vi "convert_FIFO_data_USB7855R.vi"(0 "Actual Data":i16[](array[numeric]), 5 "Calinbration Costants":cluster{"LSB Weight":u32, "Offset":i32}[](array[cluster])) -> (19 "appended array":dbl[][](array[numeric]))   [LabVIEW 2023]
uses:
  User_Vi/Settings.vi
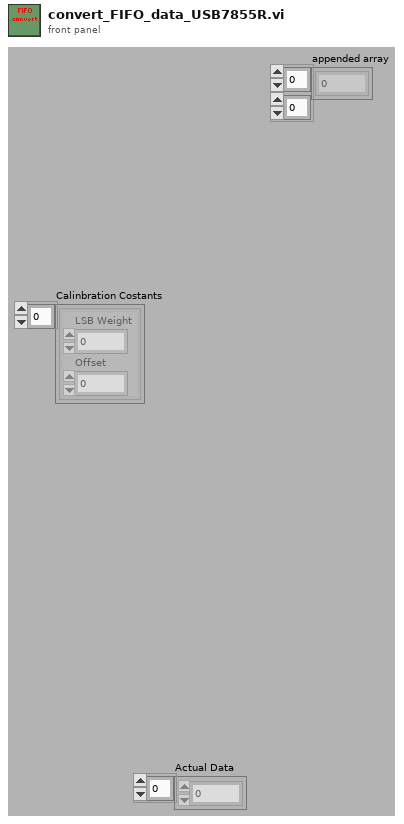
[diagram p1: front panel]
types:
  T1 = typedef "Current Amplifier Settings.ctl" = dbl
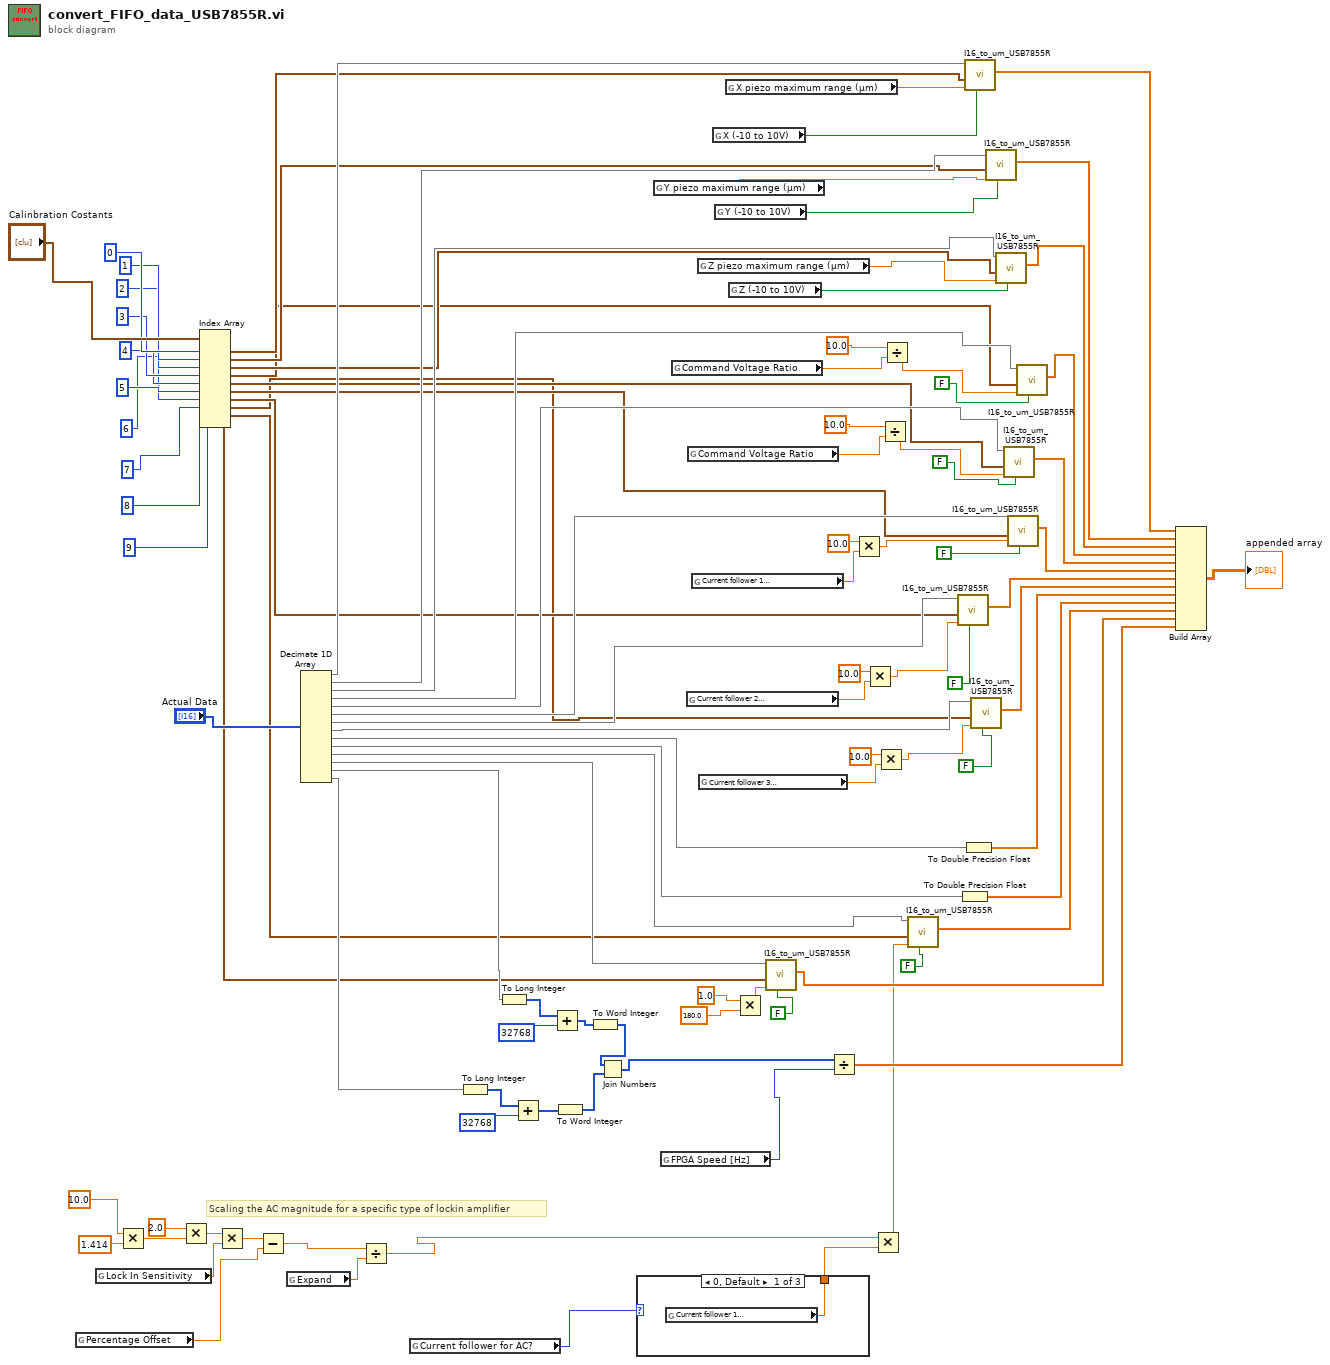
[diagram p0: block diagram]
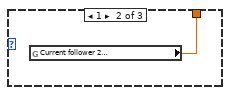
[diagram p2: hidden frame]
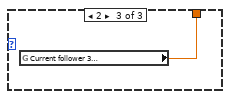
[diagram p3: hidden frame]
diagram:
  # "Scaling the AC magnitude for a specific type of lockin amplifier"
  n1 = global read "Settings.vi" "Percentage Offset"() -> (w33:dbl)
  n2 = global read "Settings.vi" "Lock In Sensitivity"() -> (w31:dbl)
  n3 = Multiply(x=10.0 ("y"), y=1.414) -> (x*y=w25:dbl)
  n4 = Multiply(x=2.0 ("y"), y=w25) -> (x*y=w30:dbl)
  n5 = Index Array(array="Calinbration Costants", index #1=0 ("index"), index #2=1 ("index"), index #3=2 ("index"), index #4=3 ("index"), index #5=4 ("index"), index #6=5 ("index"), index #7=6 ("index"), index #8=7 ("index"), index #9=8 ("index"), index #10=9 ("index")) -> (element #1=w19:cluster{"LSB Weight":u32, "Offset":i32}, element #2=w17:cluster{"LSB Weight":u32, "Offset":i32}, element #3=w10:cluster{"LSB Weight":u32, "Offset":i32}, element #4=w7:cluster{"LSB Weight":u32, "Offset":i32}, element #5=w6:cluster{"LSB Weight":u32, "Offset":i32}, element #6=w5:cluster{"LSB Weight":u32, "Offset":i32}, element #7=w4:cluster{"LSB Weight":u32, "Offset":i32}, element #8=w3:cluster{"LSB Weight":u32, "Offset":i32}, element #9=w2:cluster{"LSB Weight":u32, "Offset":i32}, element #10=w1:cluster{"LSB Weight":u32, "Offset":i32})
  n6 = Multiply(x=w30, y=w31) -> (x*y=w32:dbl)
  n7 = Subtract(x=w32, y=w33) -> (x-y=w27:dbl)
  n8 = global read "Settings.vi" "Expand"() -> (w28:dbl)
  n9 = Decimate 1D Array("Actual Data") -> (w74:i16[], w70:i16[], w64:i16[], w61:i16[], w56:i16[], w53:i16[], w49:i16[], w46:i16[], w95:i16[], w94:i16[], w37:i16[], w42:i16[], w89:i16[], w84:i16[])
  n10 = Divide(x=w27, y=w28) -> (x/y=w29:dbl)
  n11 = global read "Settings.vi" "Current follower for AC?"() -> (w35:u8)
  n12 = To Long Integer(number=w84) -> (32bit integer=w85:i32[])
  n13 = To Long Integer(number=w89) -> (32bit integer=w88:i32[])
  n14 = Add(x=w85, y=32768 ("Max Value [um]")) -> (x+y=w81:i32[])
  n15 = Add(x=w88, y=32768 ("Max Value [um]")) -> (x+y=w82:i32[])
  n16 = To Word Integer(number=w81) -> (16bit integer=w80:i16[])
  n17 = To Word Integer(number=w82) -> (16bit integer=w79:i16[])
  n18 = Join Numbers(hi=w79, lo=w80) -> ((hi.lo)=w83:u32[])
  n19 = case shown="0, Default" w35 {
    tunnel: [w106 w107 w108] -> w34
    frame 0, Default {
      n20 = global read "Settings.vi" "Current follower 1\n (AI-3)"() -> (w106:T1)
    }
    frame 1 {
      n21 = global read "Settings.vi" "Current follower 2 \n(AI-4)"() -> (w107:T1)
    }
    frame 2 {
      n22 = global read "Settings.vi" "Current follower 3\n(AI-6)"() -> (w108:T1)
    }
  }
  n23 = global read "Settings.vi" "Y piezo maximum range (µm)"() -> (w69:dbl)
  n24 = global read "Settings.vi" "FPGA Speed [Hz]"() -> (w77:i64)
  n25 = global read "Settings.vi" "Command Voltage Ratio"() -> (w76:dbl)
  n26 = global read "Settings.vi" "Current follower 2 \n(AI-4)"() -> (w99:T1)
  n27 = global read "Settings.vi" "Command Voltage Ratio"() -> (w75:dbl)
  n28 = global read "Settings.vi" "Current follower 1\n (AI-3)"() -> (w101:T1)
  n29 = global read "Settings.vi" "Z piezo maximum range (µm)"() -> (w63:dbl)
  n30 = global read "Settings.vi" "Current follower 3\n(AI-6)"() -> (w96:T1)
  n31 = global read "Settings.vi" "X (-10 to 10V)"() -> (w72:bool)
  n32 = global read "Settings.vi" "Y (-10 to 10V)"() -> (w68:bool)
  n33 = global read "Settings.vi" "X piezo maximum range (µm)"() -> (w73:dbl)
  n34 = global read "Settings.vi" "Z (-10 to 10V)"() -> (w66:bool)
  n35 = Multiply(x=1.0, y=180.0) -> (x*y=w39:dbl)
  n36 = call "I16_to_um_USB7855R.vi"("-10 to 10V range?"=FALSE, "Max Value [um]"=w39, "Channel Calibration"=w1, "Input_I16"=w42) -> ("output_um"=w41:dbl[])  [unwired: 7 in]
  n37 = Divide(x=w83, y=w77) -> (x/y=w90:dbl[])
  n38 = Multiply(x=10.0 ("Max Value [um]"), y=w101) -> (x*y=w52:T1)
  n39 = Multiply(x=10.0 ("Max Value [um]"), y=w99) -> (x*y=w48:T1)
  n40 = Multiply(x=w29, y=w34) -> (x*y=w23:T1)
  n41 = Multiply(x=10.0 ("Max Value [um]"), y=w96) -> (x*y=w43:T1)
  n42 = Divide(x=10.0 ("Max Value [um]"), y=w75) -> (x/y=w55:dbl)
  n43 = Divide(x=10.0 ("Max Value [um]"), y=w76) -> (x/y=w60:dbl)
  n44 = call "I16_to_um_USB7855R.vi"("-10 to 10V range?"=FALSE, "Max Value [um]"=w23, "Channel Calibration"=w2, "Input_I16"=w37) -> ("output_um"=w38:dbl[])  [unwired: 7 in]
  n45 = call "I16_to_um_USB7855R.vi"("-10 to 10V range?"=FALSE, "Max Value [um]"=w48, "Channel Calibration"=w4, "Input_I16"=w49) -> ("output_um"=w50:dbl[])  [unwired: 7 in]
  n46 = To Double Precision Float(number=w94) -> (double precision float=w92:dbl[])
  n47 = To Double Precision Float(number=w95) -> (double precision float=w93:dbl[])
  n48 = call "I16_to_um_USB7855R.vi"("-10 to 10V range?"=w72, "Max Value [um]"=w73, "Channel Calibration"=w19, "Input_I16"=w74) -> ("output_um"=w71:dbl[])  [unwired: 7 in]
  n49 = call "I16_to_um_USB7855R.vi"("-10 to 10V range?"=FALSE, "Max Value [um]"=w43, "Channel Calibration"=w3, "Input_I16"=w46) -> ("output_um"=w45:dbl[])  [unwired: 7 in]
  n50 = call "I16_to_um_USB7855R.vi"("-10 to 10V range?"=w68, "Max Value [um]"=w69, "Channel Calibration"=w17, "Input_I16"=w70) -> ("output_um"=w67:dbl[])  [unwired: 7 in]
  n51 = call "I16_to_um_USB7855R.vi"("-10 to 10V range?"=w66, "Max Value [um]"=w63, "Channel Calibration"=w10, "Input_I16"=w64) -> ("output_um"=w65:dbl[])  [unwired: 7 in]
  n52 = call "I16_to_um_USB7855R.vi"("-10 to 10V range?"=FALSE, "Max Value [um]"=w55, "Channel Calibration"=w6, "Input_I16"=w56) -> ("output_um"=w58:dbl[])  [unwired: 7 in]
  n53 = call "I16_to_um_USB7855R.vi"("-10 to 10V range?"=FALSE, "Max Value [um]"=w52, "Channel Calibration"=w5, "Input_I16"=w53) -> ("output_um"=w54:dbl[])  [unwired: 7 in]
  n54 = call "I16_to_um_USB7855R.vi"("-10 to 10V range?"=FALSE, "Max Value [um]"=w60, "Channel Calibration"=w7, "Input_I16"=w61) -> ("output_um"=w62:dbl[])  [unwired: 7 in]
  n55 = Build Array(w71, w67, w65, w62, w58, w54, w50, w45, w93, w92, w38, w41, w90) -> (→"appended array":dbl[][])
